vi "Clear Arbitrary Waveform.vi"(8 "error in (no error)":errorcluster, 9 "Arbitrary Waveform Name":string, 10 "Clear All Waveforms? (F: Disable)":bool, 11 "VISA resource name":refnum<visa-resource-name>) -> (0 "error out":errorcluster, 3 "VISA resource name out":refnum<visa-resource-name>)   [LabVIEW 2026, in "Agilent 33XXX Series.lvlib"]
doc: "Removes a previously created arbitrary waveform from the function generator's memory.\n\nNote: because all arbitrary waveforms are stored in non-volatile memory and therefore will remain stored regardless of power-cycling, any waveforms that may contain sensitive material should be deleted after use."
uses:
  Agilent 33XXX Series.lvlib
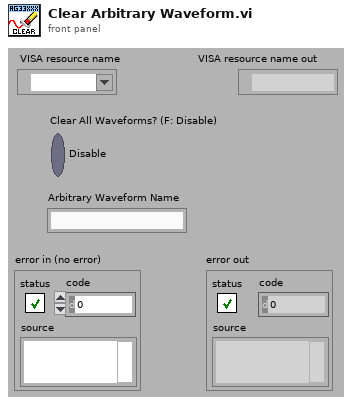
[diagram p1: front panel]
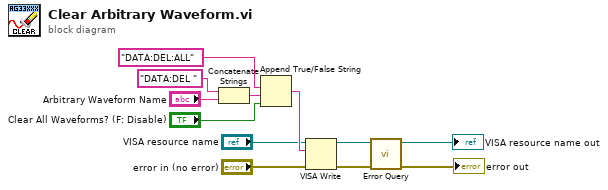
[diagram p0: block diagram]
diagram:
  n1 = Concatenate Strings("DATA:DEL " ("string"), "Arbitrary Waveform Name") -> (w8:string)
  n2 = Append True/False String(1:"Clear All Waveforms? (F: Disable)", 2:w8, 3:"DATA:DEL:ALL" ("true string")) -> (0:w6:string)  [unwired: 1 in]
  n3 = VISA Write(VISA resource name="VISA resource name", write buffer=w6, error in (no error)="error in (no error)") -> (VISA resource name out=w10:refnum<visa-resource-name>, error out=w9:errorcluster)  [unwired: 1 out]
  n4 = call "Error Query.vi"("error in (no error)"=w9, "VISA resource name"=w10) -> ("error out"=→"error out":errorcluster, "VISA resource name out"=→"VISA resource name out":refnum<visa-resource-name>)  [unwired: 6 in, 2 out]
